vi "Text-MinSec String.vi"(1 "Seconds":dbl) -> (0 "MinSec string":string)   [LabVIEW 2020]
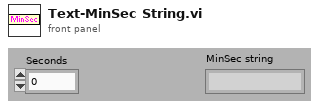
[diagram p1: front panel]
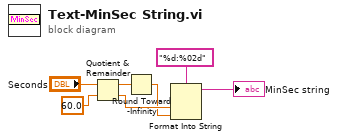
[diagram p0: block diagram]
diagram:
  n1 = Quotient & Remainder(x="Seconds", y=60.0) -> (x-y*floor(x/y)=w3:dbl, floor(x/y)=w4:dbl)
  n2 = Round Toward -Infinity(1:w3) -> (0:w1:dbl)
  n3 = Format Into String(format string="%d:%02d", w4, w1) -> (resulting string=→"MinSec string":string)  [unwired: 2 in, 1 out]
